vi "RDG822 Front Panel.vi"() -> ()   [LabVIEW 2021]
panel:
  out "error out":errorcluster
  in  "Path to \\FP":path
  in  "error in":errorcluster
  in  "VISA resource name":refnum<visa-resource-name>
  in  "PhaseDBL":dbl format="%.3f"
  in  "OK":bool
  out "Screen\nPhase":picture
  out "PhaseStr":string="5.0000"
  in  "LowL":dbl=-2.5 format="%.4f"
  in  "Offset":dbl format="%.4f"
  out "Screen\nOffset-LowL":picture
  out "Offset-LowL":string="5.0000"
  in  "Offset/LowL":bool
  in  "HighL":dbl=1.0 format="%.4f"
  in  "Ampl":dbl=5.0 format="%.4f"
  out "Screen\nAmpl-HighL":picture
  out "Ampl-HighL":string="5.0000"
  in  "Ampl/HighL":bool
  in  "Freq":dbl=1.0 format="%.10f"
  in  "Period":dbl=1.0 format="%_8g"
  out "Screen\nFreq/Period":picture
  out "Freq-Period":string="1,000000000"
  in  "Freq/Period":bool
  in  "Knob":dbl(knob) scale=0.0..10.0
  in  "Left":bool
  in  "Right":bool
  in  "Out2":bool
  in  "Out1":bool
  out "Screen":picture
  in  "Menu":bool
  in  "Home":bool
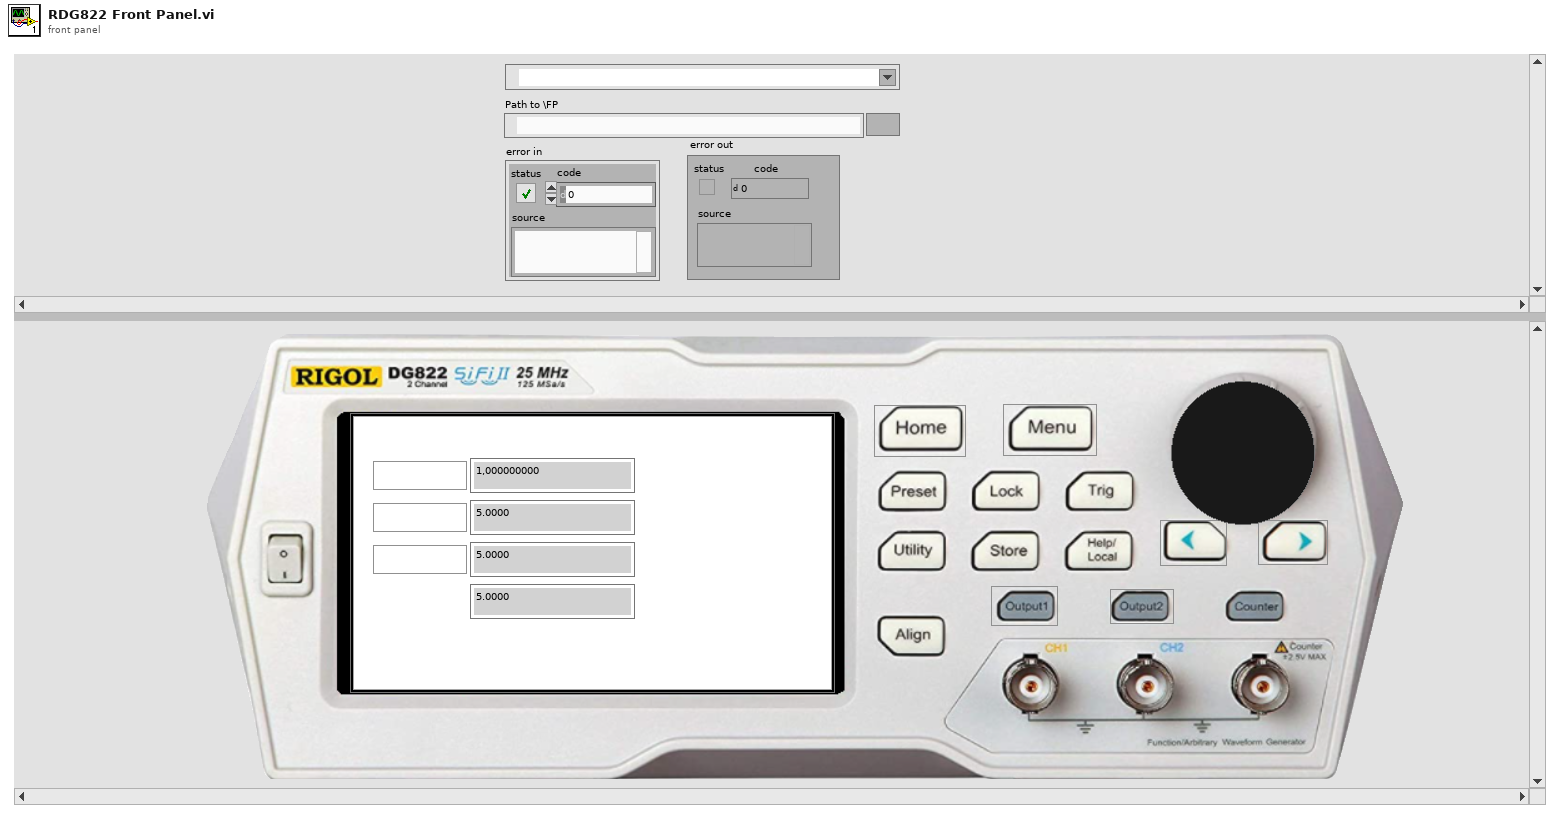
[diagram p1: front panel]
types:
  T1 = typedef "imagedata.ctl" = cluster{"image type":i32, "image depth":i32, "image":u8[], "mask":u8[], "colors":u32[], "Rectangle":cluster{"left":i16, "top":i16, "right":i16, "bottom":i16}}
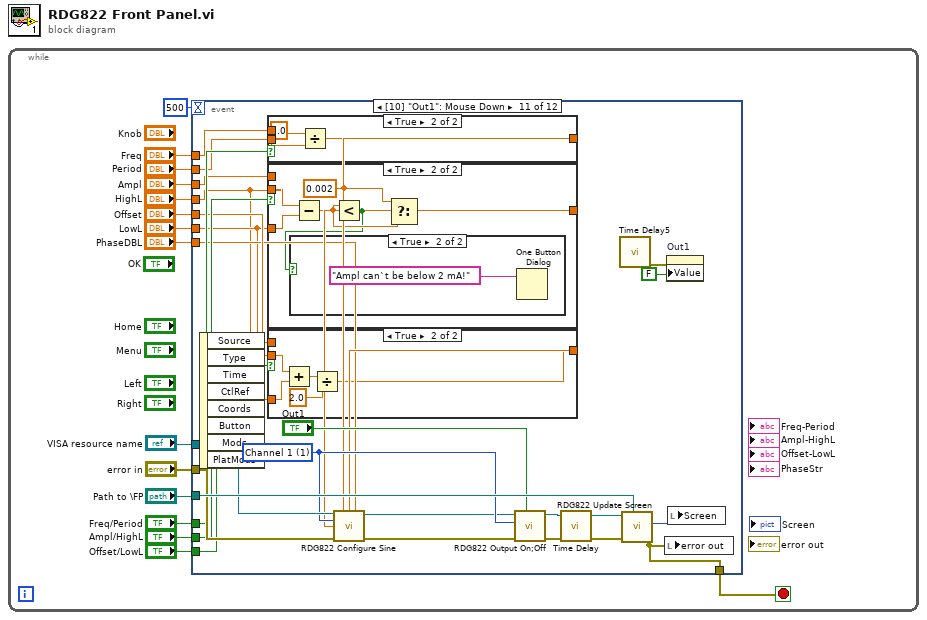
[diagram p0: block diagram]
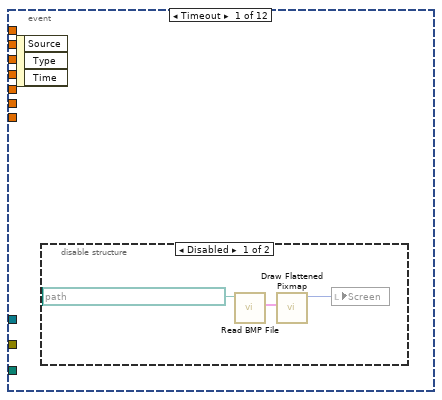
[diagram p2: hidden frame]
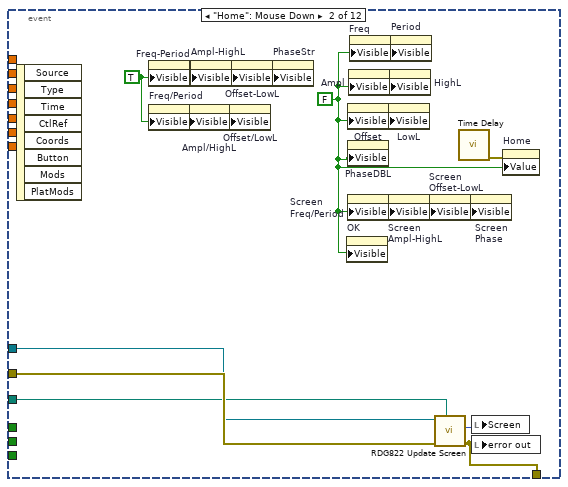
[diagram p4: hidden frame]
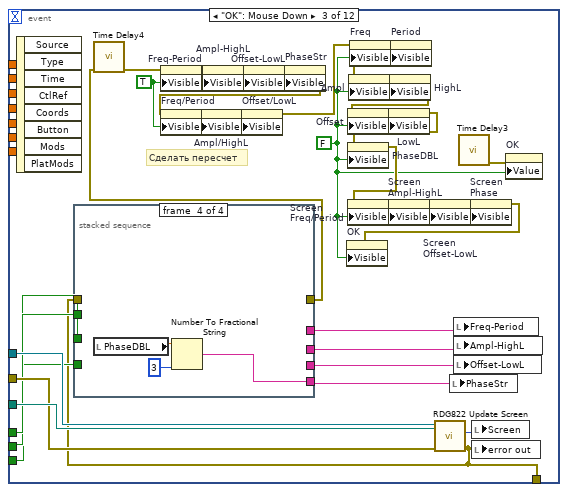
[diagram p5: hidden frame]
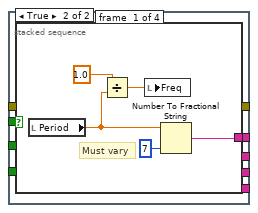
[diagram p6: hidden frame]
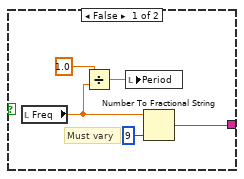
[diagram p7: hidden frame]
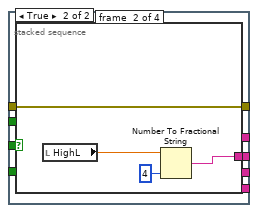
[diagram p8: hidden frame]
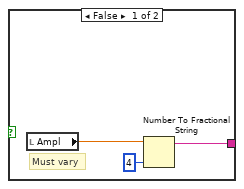
[diagram p9: hidden frame]
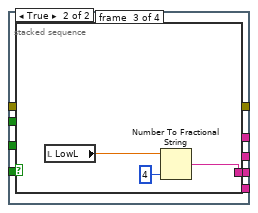
[diagram p10: hidden frame]
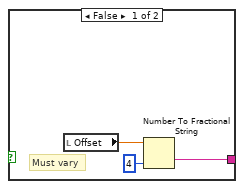
[diagram p11: hidden frame]
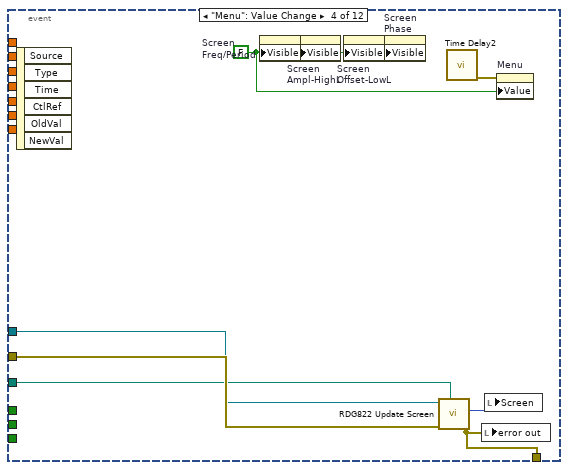
[diagram p12: hidden frame]
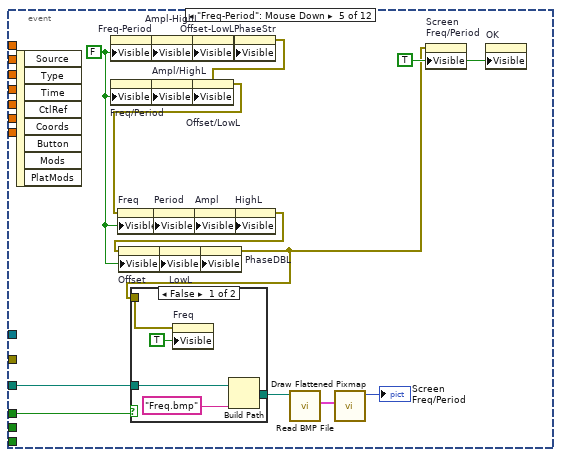
[diagram p13: hidden frame]
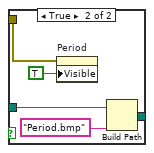
[diagram p14: hidden frame]
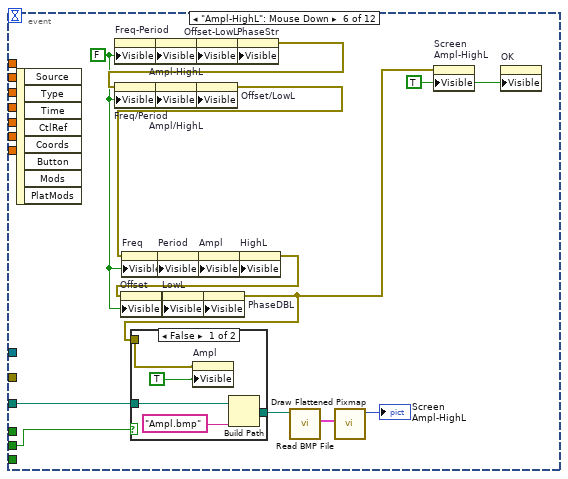
[diagram p15: hidden frame]
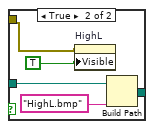
[diagram p16: hidden frame]
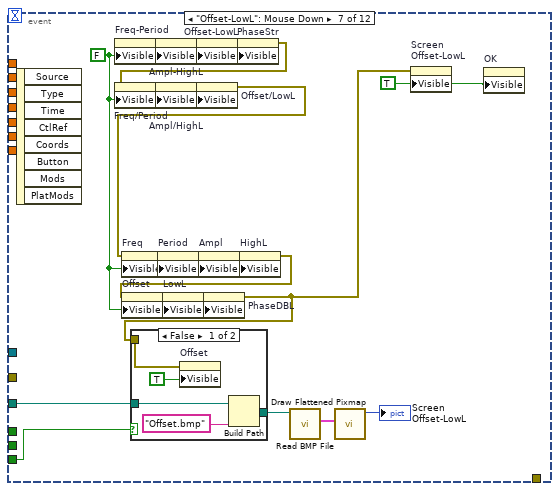
[diagram p17: hidden frame]
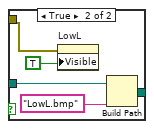
[diagram p18: hidden frame]
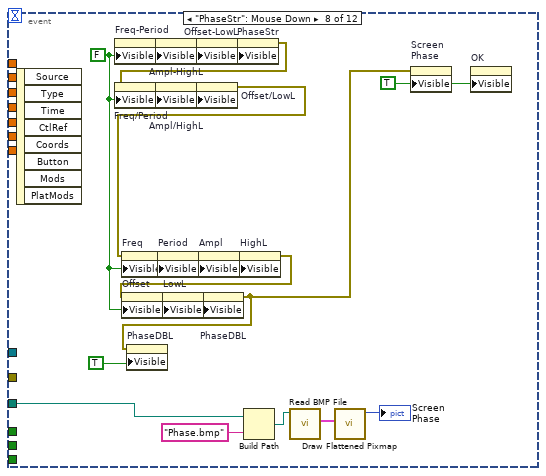
[diagram p19: hidden frame]
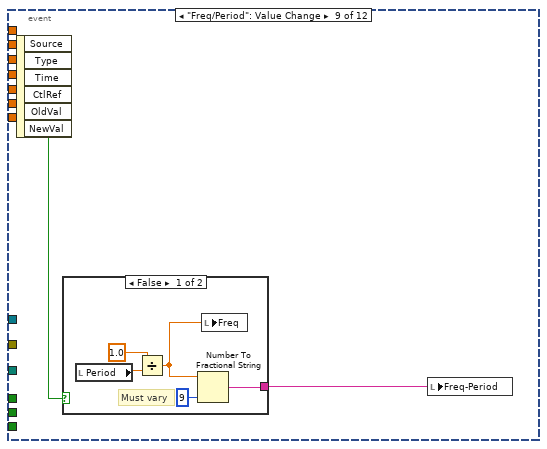
[diagram p20: hidden frame]
diagram:
  n1 = while {
    stop <- w15 stop-if-true
    n2 = event shown="[10] \"Out1\": Mouse Down" {
      selector: _ -> [_ _ _ _ _ _ _ _ _ _ _ _]
      dyn-events: _ -> [_ _ _ _ _ _ _ _ _ _ _ _]
      timeout: 500 -> [_ _ _ _ _ _ _ _ _ _ _ _]
      tunnel: [_ w25 w28 w99 _ _ _ _ _ _ w270 w302] -> w15
      tunnel: "error in" -> [_ w24 w33 w98 _ _ _ _ _ _ w264 w294]
      tunnel: "VISA resource name" -> [_ w23 w60 w97 _ _ _ _ _ _ w263 w299]
      tunnel: "Path to \\FP" -> [_ w22 w59 w96 w119 w150 w182 w199 _ _ w269 w301]
      tunnel: "Freq/Period" -> [_ _ w32 _ w117 _ _ _ _ _ w260 _]
      tunnel: "Ampl/HighL" -> [_ _ w31 _ _ w144 _ _ _ _ w261 _]
      tunnel: "Freq" -> [_ _ _ _ _ _ _ _ _ _ w259 _]
      tunnel: "Ampl" -> [_ _ _ _ _ _ _ _ _ _ w257 _]
      tunnel: "Period" -> [_ _ _ _ _ _ _ _ _ _ w258 _]
      tunnel: "HighL" -> [_ _ _ _ _ _ _ _ _ _ w247 _]
      tunnel: "Offset/LowL" -> [_ _ w30 _ _ _ w167 _ _ _ w251 _]
      tunnel: "Offset" -> [_ _ _ _ _ _ _ _ _ _ w250 _]
      tunnel: "LowL" -> [_ _ _ _ _ _ _ _ _ _ w248 _]
      tunnel: "PhaseDBL" -> [_ _ _ _ _ _ _ _ _ _ w249 _]
      event Timeout {
        n3 = event-data() -> ()  [unwired: 1 in, 3 out]
        n4 = disable-structure shown="Disabled" {
          frame Disabled {
            n5 = call <vilib>:"Read BMP File.vi"("path to BMP file"=path "E:/Study/НИР_Маг/Screen.bmp") -> ("image data"=w18:T1)  [unwired: 8 in, 2 out]
            n6 = call <vilib>:"Draw Flattened Pixmap.vi"("image data"=w18) -> ("new picture"=w16:picture)  [unwired: 8 in]
            n7 = local write "Screen"(w16) -> ()
          }
          frame Enabled {
          }
        }
      }
      event "Home": Mouse Down {
        w20 = TRUE ("Visible")
        w19 = FALSE ("Visible")
        n8 = event-data() -> ()  [unwired: 1 in, 8 out]
        n9 = property on="Freq-Period" class="Str"("Visible"=w20) -> ()  [unwired: 2 in, 2 out]
        n10 = property on="Freq/Period" class="Bool (strict)"("Visible"=w20) -> ()  [unwired: 2 in, 2 out]
        n11 = property on="Ampl/HighL" class="Bool (strict)"("Visible"=w20) -> ()  [unwired: 2 in, 2 out]
        n12 = property on="Ampl-HighL" class="Str"("Visible"=w20) -> ()  [unwired: 2 in, 2 out]
        n13 = property on="Offset/LowL" class="Bool (strict)"("Visible"=w20) -> ()  [unwired: 2 in, 2 out]
        n14 = property on="Offset-LowL" class="Str"("Visible"=w20) -> ()  [unwired: 2 in, 2 out]
        n15 = property on="PhaseStr" class="Str"("Visible"=w20) -> ()  [unwired: 2 in, 2 out]
        n16 = property on="OK" class="Bool (strict)"("Visible"=w19) -> ()  [unwired: 2 in, 2 out]
        n17 = property on="Offset" class="DigNum (strict)"("Visible"=w19) -> ()  [unwired: 2 in, 2 out]
        n18 = property on="PhaseDBL" class="DigNum (strict)"("Visible"=w19) -> ()  [unwired: 2 in, 2 out]
        n19 = property on="Screen\nFreq/Period" class="Pict"("Visible"=w19) -> ()  [unwired: 2 in, 2 out]
        n20 = property on="Ampl" class="DigNum (strict)"("Visible"=w19) -> ()  [unwired: 2 in, 2 out]
        n21 = property on="Freq" class="DigNum (strict)"("Visible"=w19) -> ()  [unwired: 2 in, 2 out]
        n22 = property on="LowL" class="DigNum (strict)"("Visible"=w19) -> ()  [unwired: 2 in, 2 out]
        n23 = property on="Screen\nAmpl-HighL" class="Pict"("Visible"=w19) -> ()  [unwired: 2 in, 2 out]
        n24 = property on="HighL" class="DigNum (strict)"("Visible"=w19) -> ()  [unwired: 2 in, 2 out]
        n25 = property on="Period" class="DigNum (strict)"("Visible"=w19) -> ()  [unwired: 2 in, 2 out]
        n26 = property on="Screen\nOffset-LowL" class="Pict"("Visible"=w19) -> ()  [unwired: 2 in, 2 out]
        n27 = call "RDG822 Update Screen.vi"("Path"=w22, "error in"=w24, "VISA resource name"=w23) -> ("error out"=w25:errorcluster, "Screen"=w26:picture)  [unwired: 7 in]
        n28 = call "Time Delay"() -> ("error out"=w21:errorcluster)  [unwired: 11 in]
        n29 = property on="Screen\nPhase" class="Pict"("Visible"=w19) -> ()  [unwired: 2 in, 2 out]
        n30 = local write "Screen"(w26) -> ()
        n31 = local write "error out"(w25) -> ()
        n32 = property on="Home" class="Bool (strict)"(error in=w21, "Value"=w19) -> ()  [unwired: 1 in, 2 out]
      }
      event "OK": Mouse Down {
        w57 = TRUE ("Visible")
        w37 = FALSE ("Visible")
        # "Сделать пересчет"
        n33 = event-data() -> ()  [unwired: 1 in, 8 out]
        n34 = call "RDG822 Update Screen.vi"("Path"=w59, "error in"=w33, "VISA resource name"=w60) -> ("error out"=w28:errorcluster, "Screen"=w61:picture)  [unwired: 7 in]
        n35 = stacked-sequence {
          tunnel: [_ _ w84 _] -> w36
          tunnel: [_ w76 _ _] -> w35
          tunnel: [w63 _ _ _] -> w34
          tunnel: w32 -> [w62 _ _ _]
          tunnel: w31 -> [_ w75 _ _]
          tunnel: w30 -> [_ _ w83 _]
          tunnel: [_ w74 _ _] -> w29
          tunnel: w28 -> [_ w74 _ _]
          tunnel: [_ _ _ w91] -> w27
          frame #0 {
            n36 = case shown="True" w62 {
              tunnel: [w68 w73] -> w63
              frame False {
                # "Must vary"
                n37 = local read "Freq"() -> (w65:dbl)
                n38 = Divide(x=1.0, y=w65) -> (x/y=w64:dbl)
                n39 = local write "Period"(w64) -> ()
                n40 = Number To Fractional String(number=w65, precision (6)=i16 9) -> (F-format string=w68:string)  [unwired: 2 in]
              }
              frame True {
                # "Must vary"
                n41 = local read "Period"() -> (w70:dbl)
                n42 = Divide(x=1.0, y=w70) -> (x/y=w69:dbl)
                n43 = local write "Freq"(w69) -> ()
                n44 = Number To Fractional String(number=w70, precision (6)=i16 7) -> (F-format string=w73:string)  [unwired: 2 in]
              }
            }
          }
          frame #1 {
            n45 = case shown="True" w75 {
              tunnel: [w78 w80] -> w76
              frame False {
                # "Must vary"
                n46 = local read "Ampl"() -> (w77:dbl)
                n47 = Number To Fractional String(number=w77, precision (6)=i16 4) -> (F-format string=w78:string)  [unwired: 2 in]
              }
              frame True {
                n48 = local read "HighL"() -> (w81:dbl)
                n49 = Number To Fractional String(number=w81, precision (6)=i16 4) -> (F-format string=w80:string)  [unwired: 2 in]
              }
            }
          }
          frame #2 {
            n50 = case shown="True" w83 {
              tunnel: [w86 w90] -> w84
              frame False {
                # "Must vary"
                n51 = local read "Offset"() -> (w87:dbl)
                n52 = Number To Fractional String(number=w87, precision (6)=i16 4) -> (F-format string=w86:string)  [unwired: 2 in]
              }
              frame True {
                n53 = local read "LowL"() -> (w88:dbl)
                n54 = Number To Fractional String(number=w88, precision (6)=i16 4) -> (F-format string=w90:string)  [unwired: 2 in]
              }
            }
          }
          frame #3 {
            n55 = local read "PhaseDBL"() -> (w93:dbl)
            n56 = Number To Fractional String(number=w93, precision (6)=i16 3) -> (F-format string=w91:string)  [unwired: 2 in]
          }
        }
        n57 = call "Time Delay4"("error in (no error)"=w29) -> ("error out"=w56:errorcluster)  [unwired: 10 in]
        n58 = property on="Freq-Period" class="Str"(error in=w56, "Visible"=w57) -> (error out=w55:errorcluster)  [unwired: 1 in, 1 out]
        n59 = property on="Ampl-HighL" class="Str"(error in=w55, "Visible"=w57) -> (error out=w54:errorcluster)  [unwired: 1 in, 1 out]
        n60 = property on="Offset-LowL" class="Str"(error in=w54, "Visible"=w57) -> (error out=w53:errorcluster)  [unwired: 1 in, 1 out]
        n61 = property on="PhaseStr" class="Str"(error in=w53, "Visible"=w57) -> (error out=w52:errorcluster)  [unwired: 1 in, 1 out]
        n62 = property on="Freq/Period" class="Bool (strict)"(error in=w52, "Visible"=w57) -> (error out=w51:errorcluster)  [unwired: 1 in, 1 out]
        n63 = property on="Ampl/HighL" class="Bool (strict)"(error in=w51, "Visible"=w57) -> (error out=w50:errorcluster)  [unwired: 1 in, 1 out]
        n64 = property on="Offset/LowL" class="Bool (strict)"(error in=w50, "Visible"=w57) -> (error out=w49:errorcluster)  [unwired: 1 in, 1 out]
        n65 = property on="Freq" class="DigNum (strict)"(error in=w49, "Visible"=w37) -> (error out=w48:errorcluster)  [unwired: 1 in, 1 out]
        n66 = property on="Period" class="DigNum (strict)"(error in=w48, "Visible"=w37) -> (error out=w47:errorcluster)  [unwired: 1 in, 1 out]
        n67 = property on="Ampl" class="DigNum (strict)"(error in=w47, "Visible"=w37) -> (error out=w46:errorcluster)  [unwired: 1 in, 1 out]
        n68 = property on="HighL" class="DigNum (strict)"(error in=w46, "Visible"=w37) -> (error out=w45:errorcluster)  [unwired: 1 in, 1 out]
        n69 = property on="Offset" class="DigNum (strict)"(error in=w45, "Visible"=w37) -> (error out=w44:errorcluster)  [unwired: 1 in, 1 out]
        n70 = property on="LowL" class="DigNum (strict)"(error in=w44, "Visible"=w37) -> (error out=w39:errorcluster)  [unwired: 1 in, 1 out]
        n71 = property on="PhaseDBL" class="DigNum (strict)"(error in=w39, "Visible"=w37) -> (error out=w38:errorcluster)  [unwired: 1 in, 1 out]
        n72 = property on="Screen\nFreq/Period" class="Pict"(error in=w38, "Visible"=w37) -> (error out=w43:errorcluster)  [unwired: 1 in, 1 out]
        n73 = property on="Screen\nAmpl-HighL" class="Pict"(error in=w43, "Visible"=w37) -> (error out=w42:errorcluster)  [unwired: 1 in, 1 out]
        n74 = property on="Screen\nOffset-LowL" class="Pict"(error in=w42, "Visible"=w37) -> (error out=w41:errorcluster)  [unwired: 1 in, 1 out]
        n75 = local write "PhaseStr"(w27) -> ()
        n76 = local write "Freq-Period"(w34) -> ()
        n77 = local write "Ampl-HighL"(w35) -> ()
        n78 = local write "Offset-LowL"(w36) -> ()
        n79 = call "Time Delay3"() -> ("error out"=w58:errorcluster)  [unwired: 11 in]
        n80 = property on="Screen\nPhase" class="Pict"(error in=w41, "Visible"=w37) -> (error out=w40:errorcluster)  [unwired: 1 in, 1 out]
        n81 = property on="OK" class="Bool (strict)"(error in=w40, "Visible"=w37) -> ()  [unwired: 1 in, 2 out]
        n82 = local write "Screen"(w61) -> ()
        n83 = local write "error out"(w28) -> ()
        n84 = property on="OK" class="Bool (strict)"(error in=w58, "Value"=w37) -> ()  [unwired: 1 in, 2 out]
      }
      event "Menu": Value Change {
        w94 = FALSE ("Visible")
        n85 = event-data() -> ()  [unwired: 1 in, 6 out]
        n86 = property on="Screen\nFreq/Period" class="Pict"("Visible"=w94) -> ()  [unwired: 2 in, 2 out]
        n87 = property on="Screen\nAmpl-HighL" class="Pict"("Visible"=w94) -> ()  [unwired: 2 in, 2 out]
        n88 = property on="Screen\nOffset-LowL" class="Pict"("Visible"=w94) -> ()  [unwired: 2 in, 2 out]
        n89 = property on="Screen\nPhase" class="Pict"("Visible"=w94) -> ()  [unwired: 2 in, 2 out]
        n90 = call "RDG822 Update Screen.vi"("Path"=w96, "error in"=w98, "VISA resource name"=w97) -> ("error out"=w99:errorcluster, "Screen"=w100:picture)  [unwired: 7 in]
        n91 = call "Time Delay2"() -> ("error out"=w95:errorcluster)  [unwired: 11 in]
        n92 = local write "error out"(w99) -> ()
        n93 = local write "Screen"(w100) -> ()
        n94 = property on="Menu" class="Bool (strict)"(error in=w95, "Value"=w94) -> ()  [unwired: 1 in, 2 out]
      }
      event "Freq-Period": Mouse Down {
        w104 = TRUE ("Visible")
        w102 = FALSE ("Visible")
        n95 = event-data() -> ()  [unwired: 1 in, 8 out]
        n96 = property on="Freq-Period" class="Str"("Visible"=w102) -> (error out=w115:errorcluster)  [unwired: 2 in, 1 out]
        n97 = property on="Ampl-HighL" class="Str"(error in=w115, "Visible"=w102) -> (error out=w111:errorcluster)  [unwired: 1 in, 1 out]
        n98 = property on="Offset-LowL" class="Str"(error in=w111, "Visible"=w102) -> (error out=w106:errorcluster)  [unwired: 1 in, 1 out]
        n99 = property on="PhaseStr" class="Str"(error in=w106, "Visible"=w102) -> (error out=w105:errorcluster)  [unwired: 1 in, 1 out]
        n100 = property on="Freq/Period" class="Bool (strict)"(error in=w105, "Visible"=w102) -> (error out=w114:errorcluster)  [unwired: 1 in, 1 out]
        n101 = property on="Ampl/HighL" class="Bool (strict)"(error in=w114, "Visible"=w102) -> (error out=w110:errorcluster)  [unwired: 1 in, 1 out]
        n102 = property on="Offset/LowL" class="Bool (strict)"(error in=w110, "Visible"=w102) -> (error out=w109:errorcluster)  [unwired: 1 in, 1 out]
        n103 = property on="Freq" class="DigNum (strict)"(error in=w109, "Visible"=w102) -> (error out=w118:errorcluster)  [unwired: 1 in, 1 out]
        n104 = property on="Period" class="DigNum (strict)"(error in=w118, "Visible"=w102) -> (error out=w113:errorcluster)  [unwired: 1 in, 1 out]
        n105 = property on="Ampl" class="DigNum (strict)"(error in=w113, "Visible"=w102) -> (error out=w112:errorcluster)  [unwired: 1 in, 1 out]
        n106 = property on="HighL" class="DigNum (strict)"(error in=w112, "Visible"=w102) -> (error out=w108:errorcluster)  [unwired: 1 in, 1 out]
        n107 = property on="Offset" class="DigNum (strict)"(error in=w108, "Visible"=w102) -> (error out=w107:errorcluster)  [unwired: 1 in, 1 out]
        n108 = property on="LowL" class="DigNum (strict)"(error in=w107, "Visible"=w102) -> (error out=w103:errorcluster)  [unwired: 1 in, 1 out]
        n109 = property on="PhaseDBL" class="DigNum (strict)"(error in=w103, "Visible"=w102) -> (error out=w101:errorcluster)  [unwired: 1 in, 1 out]
        n110 = case shown="False" w117 {
          tunnel: [w126 w131] -> w116
          tunnel: w119 -> [w124 w129]
          tunnel: w101 -> [w122 w127]
          frame False {
            n111 = property on="Freq" class="DigNum (strict)"(error in=w122, "Visible"=TRUE) -> ()  [unwired: 1 in, 2 out]
            n112 = Build Path(base path=w124, name or relative path="Freq.bmp") -> (appended path=w126:path)
          }
          frame True {
            n113 = property on="Period" class="DigNum (strict)"(error in=w127, "Visible"=TRUE) -> ()  [unwired: 1 in, 2 out]
            n114 = Build Path(base path=w129, name or relative path="Period.bmp") -> (appended path=w131:path)
          }
        }
        n115 = call <vilib>:"Read BMP File.vi"("path to BMP file"=w116) -> ("image data"=w120:T1)  [unwired: 8 in, 2 out]
        n116 = call <vilib>:"Draw Flattened Pixmap.vi"("image data"=w120) -> ("new picture"=→"Screen\nFreq/Period":picture)  [unwired: 8 in]
        n117 = property on="Screen\nFreq/Period" class="Pict"(error in=w101, "Visible"=w104) -> ()  [unwired: 1 in, 2 out]
        n118 = property on="OK" class="Bool (strict)"("Visible"=w104) -> ()  [unwired: 2 in, 2 out]
      }
      event "Ampl-HighL": Mouse Down {
        w133 = FALSE ("Visible")
        w135 = TRUE ("Visible")
        n119 = event-data() -> ()  [unwired: 1 in, 8 out]
        n120 = property on="Freq-Period" class="Str"("Visible"=w133) -> (error out=w147:errorcluster)  [unwired: 2 in, 1 out]
        n121 = property on="Ampl-HighL" class="Str"(error in=w147, "Visible"=w133) -> (error out=w142:errorcluster)  [unwired: 1 in, 1 out]
        n122 = property on="Offset-LowL" class="Str"(error in=w142, "Visible"=w133) -> (error out=w137:errorcluster)  [unwired: 1 in, 1 out]
        n123 = property on="PhaseStr" class="Str"(error in=w137, "Visible"=w133) -> (error out=w136:errorcluster)  [unwired: 1 in, 1 out]
        n124 = property on="Freq/Period" class="Bool (strict)"(error in=w136, "Visible"=w133) -> (error out=w146:errorcluster)  [unwired: 1 in, 1 out]
        n125 = property on="Ampl/HighL" class="Bool (strict)"(error in=w146, "Visible"=w133) -> (error out=w141:errorcluster)  [unwired: 1 in, 1 out]
        n126 = property on="Offset/LowL" class="Bool (strict)"(error in=w141, "Visible"=w133) -> (error out=w140:errorcluster)  [unwired: 1 in, 1 out]
        n127 = property on="Freq" class="DigNum (strict)"(error in=w140, "Visible"=w133) -> (error out=w148:errorcluster)  [unwired: 1 in, 1 out]
        n128 = property on="Period" class="DigNum (strict)"(error in=w148, "Visible"=w133) -> (error out=w145:errorcluster)  [unwired: 1 in, 1 out]
        n129 = property on="Ampl" class="DigNum (strict)"(error in=w145, "Visible"=w133) -> (error out=w143:errorcluster)  [unwired: 1 in, 1 out]
        n130 = property on="HighL" class="DigNum (strict)"(error in=w143, "Visible"=w133) -> (error out=w139:errorcluster)  [unwired: 1 in, 1 out]
        n131 = property on="Offset" class="DigNum (strict)"(error in=w139, "Visible"=w133) -> (error out=w138:errorcluster)  [unwired: 1 in, 1 out]
        n132 = property on="LowL" class="DigNum (strict)"(error in=w138, "Visible"=w133) -> (error out=w134:errorcluster)  [unwired: 1 in, 1 out]
        n133 = property on="PhaseDBL" class="DigNum (strict)"(error in=w134, "Visible"=w133) -> (error out=w132:errorcluster)  [unwired: 1 in, 1 out]
        n134 = case shown="False" w144 {
          tunnel: [w157 w162] -> w149
          tunnel: w150 -> [w155 w160]
          tunnel: w132 -> [w153 w159]
          frame False {
            n135 = property on="Ampl" class="DigNum (strict)"(error in=w153, "Visible"=TRUE) -> ()  [unwired: 1 in, 2 out]
            n136 = Build Path(base path=w155, name or relative path="Ampl.bmp") -> (appended path=w157:path)
          }
          frame True {
            n137 = property on="HighL" class="DigNum (strict)"(error in=w159, "Visible"=TRUE) -> ()  [unwired: 1 in, 2 out]
            n138 = Build Path(base path=w160, name or relative path="HighL.bmp") -> (appended path=w162:path)
          }
        }
        n139 = call <vilib>:"Read BMP File.vi"("path to BMP file"=w149) -> ("image data"=w151:T1)  [unwired: 8 in, 2 out]
        n140 = call <vilib>:"Draw Flattened Pixmap.vi"("image data"=w151) -> ("new picture"=→"Screen\nAmpl-HighL":picture)  [unwired: 8 in]
        n141 = property on="Screen\nAmpl-HighL" class="Pict"(error in=w132, "Visible"=w135) -> ()  [unwired: 1 in, 2 out]
        n142 = property on="OK" class="Bool (strict)"("Visible"=w135) -> ()  [unwired: 2 in, 2 out]
      }
      event "Offset-LowL": Mouse Down {
        w164 = FALSE ("Visible")
        w166 = TRUE ("Visible")
        n143 = event-data() -> ()  [unwired: 1 in, 8 out]
        n144 = property on="Freq-Period" class="Str"("Visible"=w164) -> (error out=w179:errorcluster)  [unwired: 2 in, 1 out]
        n145 = property on="Ampl-HighL" class="Str"(error in=w179, "Visible"=w164) -> (error out=w174:errorcluster)  [unwired: 1 in, 1 out]
        n146 = property on="Offset-LowL" class="Str"(error in=w174, "Visible"=w164) -> (error out=w169:errorcluster)  [unwired: 1 in, 1 out]
        n147 = property on="PhaseStr" class="Str"(error in=w169, "Visible"=w164) -> (error out=w168:errorcluster)  [unwired: 1 in, 1 out]
        n148 = property on="Freq/Period" class="Bool (strict)"(error in=w168, "Visible"=w164) -> (error out=w178:errorcluster)  [unwired: 1 in, 1 out]
        n149 = property on="Ampl/HighL" class="Bool (strict)"(error in=w178, "Visible"=w164) -> (error out=w173:errorcluster)  [unwired: 1 in, 1 out]
        n150 = property on="Offset/LowL" class="Bool (strict)"(error in=w173, "Visible"=w164) -> (error out=w172:errorcluster)  [unwired: 1 in, 1 out]
        n151 = property on="Freq" class="DigNum (strict)"(error in=w172, "Visible"=w164) -> (error out=w180:errorcluster)  [unwired: 1 in, 1 out]
        n152 = property on="Period" class="DigNum (strict)"(error in=w180, "Visible"=w164) -> (error out=w177:errorcluster)  [unwired: 1 in, 1 out]
        n153 = property on="Ampl" class="DigNum (strict)"(error in=w177, "Visible"=w164) -> (error out=w176:errorcluster)  [unwired: 1 in, 1 out]
        n154 = property on="HighL" class="DigNum (strict)"(error in=w176, "Visible"=w164) -> (error out=w170:errorcluster)  [unwired: 1 in, 1 out]
        n155 = property on="Offset" class="DigNum (strict)"(error in=w170, "Visible"=w164) -> (error out=w171:errorcluster)  [unwired: 1 in, 1 out]
        n156 = property on="LowL" class="DigNum (strict)"(error in=w171, "Visible"=w164) -> (error out=w165:errorcluster)  [unwired: 1 in, 1 out]
        n157 = property on="PhaseDBL" class="DigNum (strict)"(error in=w165, "Visible"=w164) -> (error out=w163:errorcluster)  [unwired: 1 in, 1 out]
        n158 = case shown="False" w167 {
          tunnel: [w188 w193] -> w181
          tunnel: w182 -> [w186 w191]
          tunnel: w163 -> [w184 w190]
          frame False {
            n159 = property on="Offset" class="DigNum (strict)"(error in=w184, "Visible"=TRUE) -> ()  [unwired: 1 in, 2 out]
            n160 = Build Path(base path=w186, name or relative path="Offset.bmp") -> (appended path=w188:path)
          }
          frame True {
            n161 = property on="LowL" class="DigNum (strict)"(error in=w190, "Visible"=TRUE) -> ()  [unwired: 1 in, 2 out]
            n162 = Build Path(base path=w191, name or relative path="LowL.bmp") -> (appended path=w193:path)
          }
        }
        n163 = call <vilib>:"Read BMP File.vi"("path to BMP file"=w181) -> ("image data"=w183:T1)  [unwired: 8 in, 2 out]
        n164 = call <vilib>:"Draw Flattened Pixmap.vi"("image data"=w183) -> ("new picture"=→"Screen\nOffset-LowL":picture)  [unwired: 8 in]
        n165 = property on="Screen\nOffset-LowL" class="Pict"(error in=w163, "Visible"=w166) -> ()  [unwired: 1 in, 2 out]
        n166 = property on="OK" class="Bool (strict)"("Visible"=w166) -> ()  [unwired: 2 in, 2 out]
      }
      event "PhaseStr": Mouse Down {
        w196 = FALSE ("Visible")
        w198 = TRUE ("Visible")
        n167 = event-data() -> ()  [unwired: 1 in, 8 out]
        n168 = property on="Freq-Period" class="Str"("Visible"=w196) -> (error out=w213:errorcluster)  [unwired: 2 in, 1 out]
        n169 = property on="Ampl-HighL" class="Str"(error in=w213, "Visible"=w196) -> (error out=w208:errorcluster)  [unwired: 1 in, 1 out]
        n170 = property on="Offset-LowL" class="Str"(error in=w208, "Visible"=w196) -> (error out=w203:errorcluster)  [unwired: 1 in, 1 out]
        n171 = property on="PhaseStr" class="Str"(error in=w203, "Visible"=w196) -> (error out=w202:errorcluster)  [unwired: 1 in, 1 out]
        n172 = property on="Freq/Period" class="Bool (strict)"(error in=w202, "Visible"=w196) -> (error out=w212:errorcluster)  [unwired: 1 in, 1 out]
        n173 = property on="Ampl/HighL" class="Bool (strict)"(error in=w212, "Visible"=w196) -> (error out=w207:errorcluster)  [unwired: 1 in, 1 out]
        n174 = property on="Offset/LowL" class="Bool (strict)"(error in=w207, "Visible"=w196) -> (error out=w206:errorcluster)  [unwired: 1 in, 1 out]
        n175 = property on="Freq" class="DigNum (strict)"(error in=w206, "Visible"=w196) -> (error out=w214:errorcluster)  [unwired: 1 in, 1 out]
        n176 = property on="Period" class="DigNum (strict)"(error in=w214, "Visible"=w196) -> (error out=w211:errorcluster)  [unwired: 1 in, 1 out]
        n177 = property on="Ampl" class="DigNum (strict)"(error in=w211, "Visible"=w196) -> (error out=w210:errorcluster)  [unwired: 1 in, 1 out]
        n178 = property on="HighL" class="DigNum (strict)"(error in=w210, "Visible"=w196) -> (error out=w204:errorcluster)  [unwired: 1 in, 1 out]
        n179 = property on="Offset" class="DigNum (strict)"(error in=w204, "Visible"=w196) -> (error out=w205:errorcluster)  [unwired: 1 in, 1 out]
        n180 = property on="LowL" class="DigNum (strict)"(error in=w205, "Visible"=w196) -> (error out=w197:errorcluster)  [unwired: 1 in, 1 out]
        n181 = property on="PhaseDBL" class="DigNum (strict)"(error in=w197, "Visible"=w196) -> (error out=w195:errorcluster)  [unwired: 1 in, 1 out]
        n182 = property on="PhaseDBL" class="DigNum (strict)"(error in=w195, "Visible"=TRUE) -> ()  [unwired: 1 in, 2 out]
        n183 = Build Path(base path=w199, name or relative path="Phase.bmp") -> (appended path=w201:path)
        n184 = call <vilib>:"Read BMP File.vi"("path to BMP file"=w201) -> ("image data"=w215:T1)  [unwired: 8 in, 2 out]
        n185 = call <vilib>:"Draw Flattened Pixmap.vi"("image data"=w215) -> ("new picture"=→"Screen\nPhase":picture)  [unwired: 8 in]
        n186 = property on="Screen\nPhase" class="Pict"(error in=w195, "Visible"=w198) -> ()  [unwired: 1 in, 2 out]
        n187 = property on="OK" class="Bool (strict)"("Visible"=w198) -> ()  [unwired: 2 in, 2 out]
      }
      event "Freq/Period": Value Change {
        n188 = event-data() -> ("NewVal"=w216:bool)  [unwired: 1 in, 5 out]
        n189 = case shown="False" w216 {
          tunnel: [w222 w227] -> w217
          frame False {
            # "Must vary"
            n190 = local read "Period"() -> (w220:dbl)
            n191 = Divide(x=1.0, y=w220) -> (x/y=w218:dbl)
            n192 = Number To Fractional String(number=w218, precision (6)=i16 9) -> (F-format string=w222:string)  [unwired: 2 in]
            n193 = local write "Freq"(w218) -> ()
          }
          frame True {
            # "Must vary"
            n194 = local read "Freq"() -> (w224:dbl)
            n195 = Divide(x=1.0, y=w224) -> (x/y=w223:dbl)
            n196 = local write "Period"(w223) -> ()
            n197 = Number To Fractional String(number=w223, precision (6)=i16 7) -> (F-format string=w227:string)  [unwired: 2 in]
          }
        }
        n198 = local write "Freq-Period"(w217) -> ()
      }
      event "Ampl/HighL", "Offset/LowL": Value Change {
        # "Сделать пересчет"
        n199 = event-data() -> ("NewVal"=w230:bool)  [unwired: 1 in, 5 out]
        n200 = case shown="False" w230 {
          tunnel: [w234 w238] -> w231
          frame False {
            # "Must vary"
            n201 = local read "Offset"() -> (w235:dbl)
            n202 = Number To Fractional String(number=w235, precision (6)=i16 4) -> (F-format string=w234:string)  [unwired: 2 in]
          }
          frame True {
            n203 = local read "LowL"() -> (w236:dbl)
            n204 = Number To Fractional String(number=w236, precision (6)=i16 4) -> (F-format string=w238:string)  [unwired: 2 in]
          }
        }
        n205 = case shown="False" w230 {
          tunnel: [w240 w244] -> w232
          frame False {
            # "Must vary"
            n206 = local read "Ampl"() -> (w241:dbl)
            n207 = Number To Fractional String(number=w241, precision (6)=i16 4) -> (F-format string=w240:string)  [unwired: 2 in]
          }
          frame True {
            n208 = local read "HighL"() -> (w242:dbl)
            n209 = Number To Fractional String(number=w242, precision (6)=i16 4) -> (F-format string=w244:string)  [unwired: 2 in]
          }
        }
        n210 = local read "Ampl/HighL"() -> (w229:bool)
        n211 = local read "Offset/LowL"() -> (w228:bool)
        n212 = local write "Ampl-HighL"(w232) -> ()
        n213 = local write "Offset-LowL"(w231) -> ()
        n214 = local write "Offset/LowL"(w229) -> ()
        n215 = local write "Ampl/HighL"(w228) -> ()
      }
      event "Out1": Mouse Down {
        w262 = 1 items=["Channel 1"=1, "Channel 2"=2] ("Output Channel (1: Channel 1)")
        n216 = event-data() -> ()  [unwired: 1 in, 8 out]
        n217 = case shown="True" w260 {
          tunnel: w259 -> [w290 _]
          tunnel: w258 -> [_ w292]
          tunnel: [w290 w291] -> w256
          frame False {
          }
          frame True {
            n218 = Divide(x=1.0, y=w292) -> (x/y=w291:dbl)
          }
        }
        n219 = case shown="True" w261 {
          tunnel: w257 -> [w278 _]
          tunnel: w247 -> [_ w288]
          tunnel: [w280 w286] -> w255
          tunnel: w248 -> [_ w287]
          frame False {
            w281 = 0.002 ("t")
            n220 = Less?(x=w278, y=w281) -> (x < y?=w279:bool)
            n221 = case shown="True" w279 {
              frame False {
              }
              frame True {
                n222 = One Button Dialog(message="Ampl can`t be below 2 mA!") -> ()  [unwired: 1 in, 1 out]
              }
            }
            n223 = Select(t=w281, s=w279, f=w278) -> (s? t:f=w280:dbl)
          }
          frame True {
            w283 = 0.002 ("t")
            n224 = Subtract(x=w288, y=w287) -> (x-y=w285:dbl)
            n225 = Less?(x=w285, y=w283) -> (x < y?=w284:bool)
            n226 = case shown="True" w284 {
              frame False {
              }
              frame True {
                n227 = One Button Dialog(message="Ampl can`t be below 2 mA!") -> ()  [unwired: 1 in, 1 out]
              }
            }
            n228 = Select(t=w283, s=w284, f=w285) -> (s? t:f=w286:dbl)
          }
        }
        n229 = case shown="True" w251 {
          tunnel: w250 -> [w272 _]
          tunnel: w248 -> [_ w277]
          tunnel: [w272 w273] -> w252
          tunnel: w247 -> [_ w274]
          frame False {
          }
          frame True {
            n230 = Add(x=w274, y=w277) -> (x+y=w276:dbl)
            n231 = Divide(x=w276, y=2.0) -> (x/y=w273:dbl)
          }
        }
        n232 = call "RDG822 Configure Sine.vi"("VISA resource name"=w263, "Frequency (1000 Hz)"=w256, "Phase (0 Degree)"=w249, "Output Channel (1: Channel 1)"=w262, "Amplitude (5 Vpp)"=w255, "error in (no error)"=w264, "Offset (0)"=w252) -> ("VISA resource name out"=w254:refnum<visa-resource-name>, "error out"=w253:errorcluster)  [unwired: 7 in]
        n233 = call "RDG822 Output On;Off.vi"("Enable Output (T: Enable)"="Out1", "error in (no error)"=w253, "Output Channel (1: Channel 1)"=w262, "VISA resource name"=w254) -> ("error out"=w266:errorcluster, "VISA resource name out"=w268:refnum<visa-resource-name>)  [unwired: 6 in]
        n234 = call "Time Delay"("error in (no error)"=w266) -> ("error out"=w265:errorcluster)  [unwired: 10 in]
        n235 = call "Time Delay5"() -> ("error out"=w246:errorcluster)  [unwired: 11 in]
        n236 = call "RDG822 Update Screen.vi"("Path"=w269, "error in"=w265, "VISA resource name"=w268) -> ("error out"=w270:errorcluster, "Screen"=w271:picture)  [unwired: 7 in]
        n237 = local write "error out"(w270) -> ()
        n238 = property on="Out1" class="Bool (strict)"(error in=w246, "Value"=FALSE ("Out1")) -> ()  [unwired: 1 in, 2 out]
        n239 = local write "Screen"(w271) -> ()
      }
      event "Out2": Value Change {
        w300 = 2 items=["Channel 1"=1, "Channel 2"=2] ("Output Channel (1: Channel 1)")
        # "Same as Out1 eventually"
        n240 = event-data() -> ()  [unwired: 1 in, 6 out]
        n241 = call "RDG822 Output On;Off.vi"("Enable Output (T: Enable)"="Out2", "error in (no error)"=w294, "Output Channel (1: Channel 1)"=w300, "VISA resource name"=w299) -> ("error out"=w296:errorcluster, "VISA resource name out"=w298:refnum<visa-resource-name>)  [unwired: 6 in]
        n242 = call "Time Delay"("error in (no error)"=w296) -> ("error out"=w295:errorcluster)  [unwired: 10 in]
        n243 = call "RDG822 Update Screen.vi"("Path"=w301, "error in"=w295, "VISA resource name"=w298) -> ("error out"=w302:errorcluster, "Screen"=w303:picture)  [unwired: 7 in]
        n244 = local write "error out"(w302) -> ()
        n245 = local write "Screen"(w303) -> ()
      }
    }
  }
